vi "LED_Globals.vi"() -> ()   [LabVIEW 2020]
panel:
  in  "Numbers":dbl[](array[numeric])=[2.0, 4.0, 100.0, 30.0, 2.0, 6.0]
  in  "Colors":u32[](array[colorbox])=[16732482, 2626303, 7012185]
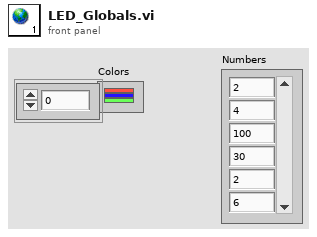
[diagram p1: front panel]
diagram:
